vi "CS SQL Client.vi"(0 "Data Source":string, 1 "Address":string="localhost", 2 "Process":string, 3 "error in (no error)":errorcluster, 4 "timeout ms (5000)":i32=5000) -> (6 "query results":string[][](array[string]), 7 "Class":string, 8 "Timeout":bool, 9 "error out":errorcluster)   [LabVIEW 2015, in "CS SQL Server.lvlib"]
doc: "This VI is the client for the CS SQL Server Application that executes the SQL request remotly."
uses:
  CS SQL Server.lvlib
  CS SQL Server Input Cluster.ctl
  CS SQL Server Output Cluster.ctl
panel:
  out "CS SQL Read Output cluster":T1
  out "CS SQL Read Input Cluster":T2 {"Version" format="%.2f"}
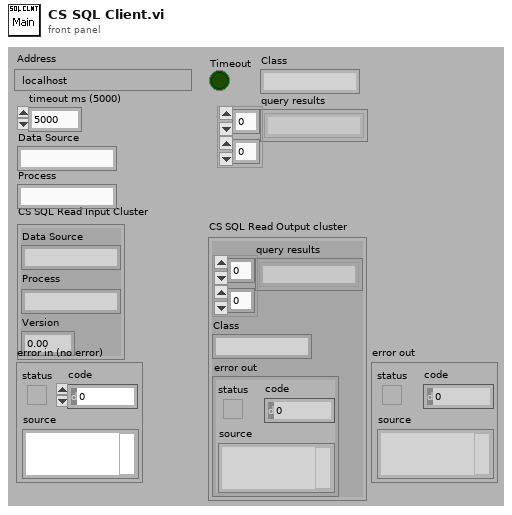
[diagram p1: front panel]
types:
  T1 = typedef "CS SQL Server.lvlib/CS SQL Server Output Cluster.ctl" = cluster{"query results":string[][], "Class":string, "error out":errorcluster}
  T2 = typedef "CS SQL Server.lvlib/CS SQL Server Input Cluster.ctl" = cluster{"Data Source":string, "Process":string, "Version":dbl}
  T3 = enum16{"connect", "disconnect", "reconnect", "default"}
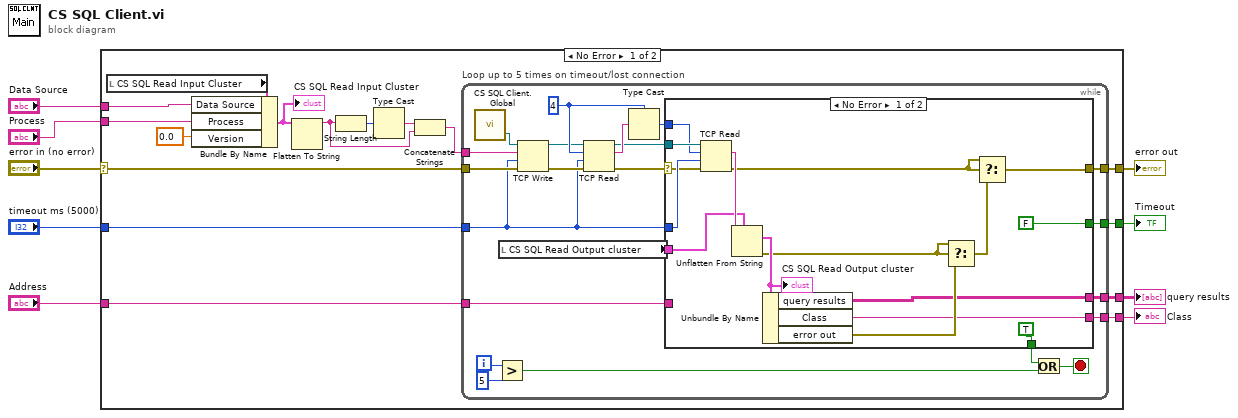
[diagram p0: block diagram]
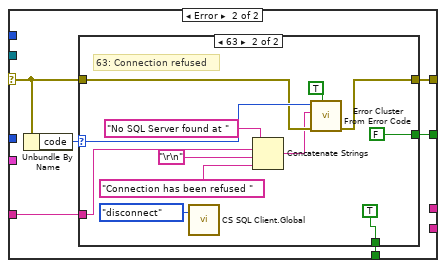
[diagram p2: hidden frame]
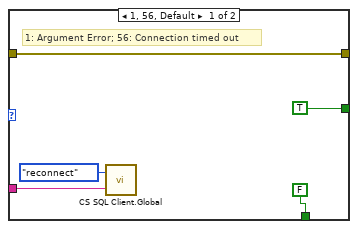
[diagram p3: hidden frame]
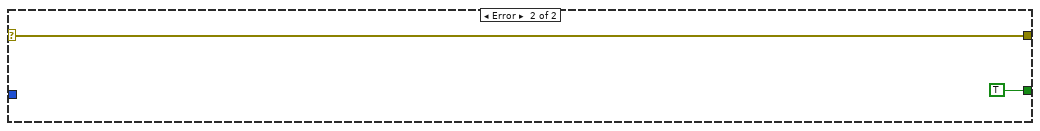
[diagram p4: hidden frame]
diagram:
  n1 = case shown="No Error" "error in (no error)" {
    selector: "error in (no error)" -> [w12 w88]
    tunnel: [w25 w88] -> w9
    tunnel: "Data Source" -> [w17 _]
    tunnel: "Process" -> [w16 _]
    tunnel: [w15 TRUE] -> w6
    tunnel: "Address" -> [w14 _]
    tunnel: "timeout ms (5000)" -> [w13 _]
    tunnel: [w11 _] -> w2
    tunnel: [w10 _] -> w1
    frame No Error {
      n2 = local read "CS SQL Read Input Cluster"() -> (w20:T2)
      n3 = Bundle By Name(cluster=w20, "Data Source"=w17, "Process"=w16, "Version"=0.0) -> (w19:T2)
      "CS SQL Read Input Cluster" <- w19
      n4 = Flatten To String(anything=w19) -> (data string=w22:string)  [unwired: 3 in, 2 out]
      n5 = String Length(string=w22) -> (length=w24:i32)
      n6 = Type Cast(x=w24) -> (*(type *) &x=w23:string)  [unwired: 1 in]
      n7 = Concatenate Strings(w23, w22) -> (w21:string)
      n8 = while "Loop up to 5 times on timeout/lost connection" {
        tunnel: [w47] -> w25
        tunnel: w21 -> [w46]
        tunnel: w12 -> [w37]
        tunnel: [w30] -> w15
        tunnel: w14 -> [w29]
        tunnel: w13 -> [w28]
        tunnel: [w27] -> w11
        tunnel: [w26] -> w10
        i -> [w34]
        stop <- w35 stop-if-true
        w44 = 4
        n9 = call "CS SQL Client.Global.vi"() -> ("connection out"=w31:refnum<k5>)  [unwired: 3 in]
        n10 = Greater?(x=w34, y=5) -> (0:w32:bool)
        n11 = local read "CS SQL Read Output cluster"() -> (w40:T1)
        n12 = TCP Write(connection ID=w31, data in=w46, error in (no error)=w37, 9:w28) -> (connection ID out=w41:refnum<k5>, error out=w42:errorcluster)  [unwired: 1 out]
        n13 = TCP Read(connection ID=w41, bytes to read=w44, error in (no error)=w42, 9:w28) -> (connection ID out=w43:refnum<k5>, data out=w45:string, error out=w38:errorcluster)  [unwired: 1 in]
        n14 = Type Cast(type=w44, x=w45) -> (*(type *) &x=w39:i32)
        n15 = case shown="No Error" w38 {
          selector: w38 -> [w53 w65]
          tunnel: w43 -> [w63 _]
          tunnel: [w59 w64] -> w47
          tunnel: w40 -> [w61 _]
          tunnel: w28 -> [w58 _]
          tunnel: w39 -> [w54 _]
          tunnel: [TRUE w68] -> w36
          tunnel: [FALSE w67] -> w30
          tunnel: w29 -> [_ w66]
          tunnel: [w49 _] -> w27
          tunnel: [w48 _] -> w26
          frame No Error {
            n16 = TCP Read(connection ID=w63, bytes to read=w54, error in (no error)=w53, 9:w58) -> (data out=w62:string, error out=w57:errorcluster)  [unwired: 1 in, 1 out]
            n17 = Unflatten From String(type=w61, binary string=w62) -> (value=w60:T1, error out=w50:errorcluster)  [unwired: 3 in, 1 out]
            "CS SQL Read Output cluster" <- w60
            n18 = Unbundle By Name(w60) -> ("query results"=w48:string[][], "Class"=w49:string, "error out"=w56:errorcluster)
            n19 = Select(t=w50, s=w50, f=w56) -> (s? t:f=w55:errorcluster)
            n20 = Select(t=w57, s=w57, f=w55) -> (s? t:f=w59:errorcluster)
          }
          frame Error {
            n21 = Unbundle By Name(w65) -> ("code"=w69:i32)
            n22 = case shown="63" w69 {
              selector: w69 -> [_ w79]
              tunnel: [FALSE TRUE] -> w68
              tunnel: [TRUE FALSE] -> w67
              tunnel: w66 -> [w71 w80]
              tunnel: w65 -> [w70 w78]
              tunnel: [w70 w77] -> w64
              frame 1, 56, Default {
                # "1: Argument Error; 56: Connection timed out"
                n23 = call "CS SQL Client.Global.vi"("Address"=w71, "command"=T3."reconnect") -> ()  [unwired: 1 in, 1 out]
              }
              frame 63 {
                # "63: Connection refused"
                n24 = call "CS SQL Client.Global.vi"("command"=T3."disconnect") -> ()  [unwired: 2 in, 1 out]
                n25 = Concatenate Strings("No SQL Server found at ", w80, "\r\n", "Connection has been refused ") -> (w76:string)
                n26 = call <vilib>:"Error Cluster From Error Code.vi"("show call chain? (False)"=TRUE, "error in (no error)"=w78, "error message (\"\")"=w76, "error code (0)"=w79) -> ("error out"=w77:errorcluster)  [unwired: 5 in]
              }
            }
          }
        }
        n27 = Or(x=w36, y=w32) -> (x .or. y?=w35:bool)
      }
    }
    frame Error {
    }
  }
  "error out" <- w9
  "Timeout" <- w6
  "Class" <- w2
  "query results" <- w1
